vi "adc2volts.vi"(1 "ADC value":u16[](array[numeric])) -> (0 "Volts":dbl[](array[numeric]))   [LabVIEW 2014]
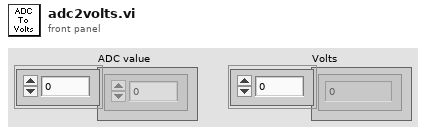
[diagram p1: front panel]
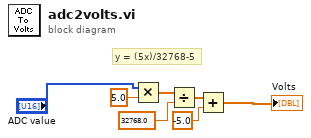
[diagram p0: block diagram]
diagram:
  # "y = (5x)/32768-5"
  n1 = Multiply(x="ADC value", y=5.0) -> (x*y=w4:dbl[])
  n2 = Divide(x=w4, y=32768.0) -> (x/y=w1:dbl[])
  n3 = Add(x=w1, y=-5.0) -> (x+y=→"Volts":dbl[])
